vi "Compute HSL Color Ranges.vi"(8 "Margins":cluster{"Hue":i32, "Sat":i32, "Lum":i32}, 9 "Luminance":i32, 10 "Saturation":i32, 11 "Hue":i32) -> (1 "Lum Range":cluster{i32, i32}, 2 "Sat Range":cluster{i32, i32}, 3 "Hue Range":cluster{i32, i32})   [LabVIEW 2015]
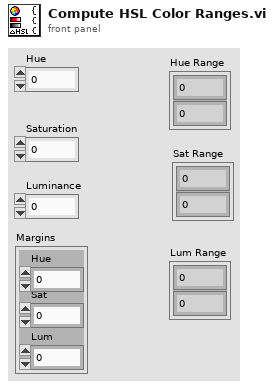
[diagram p1: front panel]
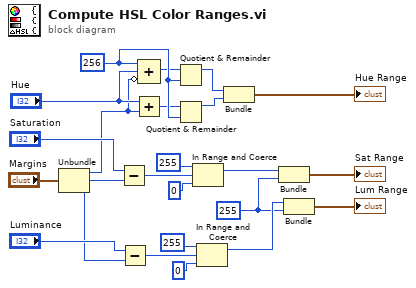
[diagram p0: block diagram]
diagram:
  w14 = 255
  w13 = 256
  n1 = Unbundle("Margins") -> ("Hue"=w6:i32, "Sat"=w5:i32, "Lum"=w4:i32)
  n2 = Subtract(x="Saturation", y=w5) -> (x-y=w17:i32)
  n3 = Subtract(x="Luminance", y=w4) -> (x-y=w21:i32)
  n4 = Add(x="Hue", y=w6) -> (x+y=w10:i32)
  n5 = Compound Arithmetic op=ADD(w13, "Hue", invert w6) -> (w11:i32)
  n6 = Quotient & Remainder(x=w11, y=w13) -> (x-y*floor(x/y)=w9:i32)  [unwired: 1 out]
  n7 = Quotient & Remainder(x=w10, y=w13) -> (x-y*floor(x/y)=w8:i32)  [unwired: 1 out]
  n8 = In Range and Coerce(upper limit=255, x=w17, lower limit=0) -> (coerced(x)=w19:i32)  [unwired: 1 out]
  n9 = In Range and Coerce(upper limit=255, x=w21, lower limit=0) -> (coerced(x)=w24:i32)  [unwired: 1 out]
  n10 = Bundle(w9, w8) -> (→"Hue Range":cluster{i32, i32})  [unwired: 1 in]
  n11 = Bundle(w19, w14) -> (→"Sat Range":cluster{i32, i32})  [unwired: 1 in]
  n12 = Bundle(w24, w14) -> (→"Lum Range":cluster{i32, i32})  [unwired: 1 in]
